vi "Check Aborted.vi"(8 "error in (no error)":errorcluster, 9 "timeout in ms (0)":i32, 11 "Slave Test Runner In":refnum<class "Slave Test Runner.lvclass">) -> (0 "error out":errorcluster, 1 "Aborted?":bool, 3 "Slave Test Runner Out":refnum<class "Slave Test Runner.lvclass">)   [LabVIEW 2020, in "Slave Test Runner.lvclass"]
doc: "Check the abort notifier."
uses:
  Slave Test Runner.lvclass
  Slave Test Runner.lvclass/Slave Test Runner.ctl
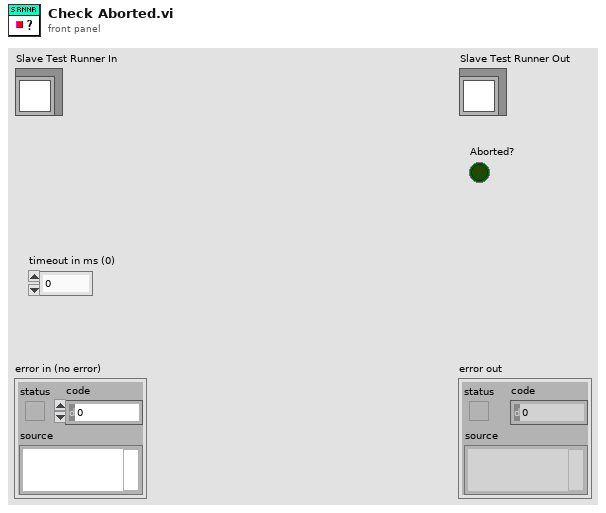
[diagram p1: front panel]
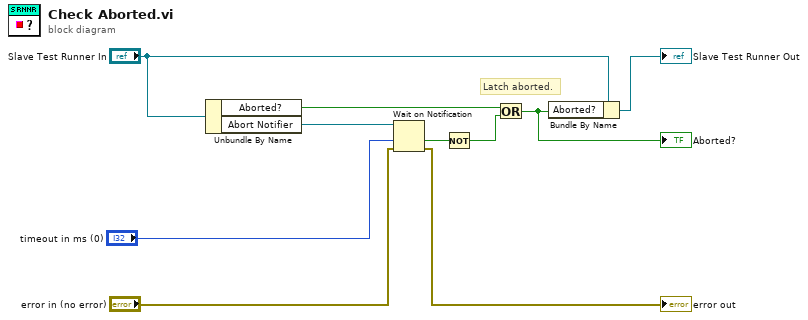
[diagram p0: block diagram]
diagram:
  # "Latch aborted."
  n1 = Unbundle By Name("Slave Test Runner In") -> ("Aborted?"=w2:bool, "Abort Notifier"=w10:refnum<notifier>)
  n2 = Wait on Notification(notifier=w10, timeout in ms (-1)="timeout in ms (0)", error in (no error)="error in (no error)") -> (timed out?=w6:bool, error out=→"error out":errorcluster)  [unwired: 1 in, 2 out]
  n3 = Not(x=w6) -> (.not. x?=w3:bool)
  n4 = Or(x=w2, y=w3) -> (x .or. y?=w1:bool)
  "Aborted?" <- w1
  n5 = Bundle By Name(cluster="Slave Test Runner In", "Aborted?"=w1) -> (→"Slave Test Runner Out":refnum<class "Slave Test Runner.lvclass">)
